vi "Read ADC To Voltage Zoom.vi"(8 "error in (no error)":errorcluster, 11 "channel":i8) -> (0 "error out":errorcluster, 3 "function return":dbl)   [LabVIEW 2021, in "vmmso.lvlib"]
doc: "DLL_API double WINAPI ReadADCToVoltageZoom(char channel);"
uses:
  vmmso.lvlib
  vmmso.dll
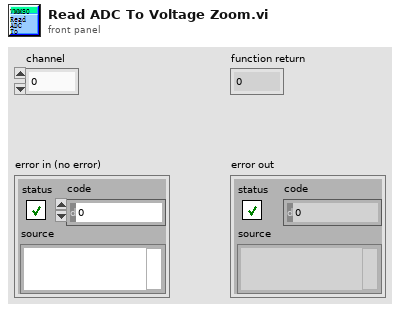
[diagram p1: front panel]
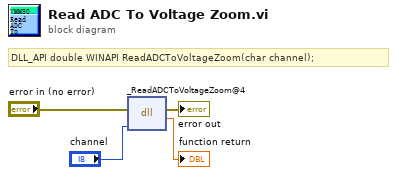
[diagram p0: block diagram]
diagram:
  # "DLL_API double WINAPI ReadADCToVoltageZoom(char channel);"
  n1 = dll-call lib="O:/MSO/library/demo-Labview/vmmso/vmmso.*" fn="_ReadADCToVoltageZoom@4"(error in="error in (no error)", "channel"="channel") -> (error out=→"error out":errorcluster, →"function return":dbl)  [unwired: 3 in, 1 out]
